vi "Identify Resource Name.vi"() -> ()   [LabVIEW 2010]
doc: "I. Description:\nThis example demonstrates how to acquire a finite amount of data (waveform) using the DAQ device's internal clock.\n\nII. Instructions for Running:\n1. Select the physical channel to correspond to where your signal is input on the DAQ device.\n2. Enter the minimum and maximum voltages.\nNote: For better accuracy try to match the input range to the expected voltage level of the measured signal.\n3. Select the number of samples to acquire.\n4. Set the rate of the acquisition\nNote: The rate should be AT LEAST twice as fast as the maximum frequency component of the signal being acquired.\n\nIII. Block Diagram Steps:\n1. Create an analog input voltage channel.\n2. Set the rate for the sample clock. Additionally, define the sample mode to be finite and set the number of samples to be acquired per channel.\n3. Call the Start VI to start the acquisition.\n4. Use the Read VI to measure multiple samples from N Channels on the device. Set a timeout so an error is returned if the samples are not returned in the specified time limit\n5. Call the Clear Task VI to clear the Task.\n6. Use the popup dialog box to display an error if any.\n \nIV. I/O Connections Overview:\nMake sure your signal input terminal matches the Physical Channel I/O Control. For further connection information, refer to your hardware reference manual."
uses:
  <vilib>/Utility/error.llb/DialogType.ctl
  <vilib>/DAQmx/read.llb/DAQmx Read (Analog 1D Wfm NChan NSamp).vi
  <vilib>/DAQmx/create/channels.llb/DAQmx Create Channel (AI-Voltage-Basic).vi
  <vilib>/DAQmx/configure/timing.llb/DAQmx Timing (Sample Clock).vi
  <vilib>/daqmx/miscellaneous.llb/DAQmx Fill In Error Info.vi
  Program Files/National Instruments/LabVIEW 2010/resource/objmgr/daqmx.rc
panel:
  in  "Desired Channels":string="/ai0:3"
  in  "ProductType you are looking for":string="PXI-4472"
  out "Physical Channels":string
  out "DAQmx Device Name":tag
  out "Array 2":string[](array[string])
  out "DevNames":tag[](array[tag])
  in  "Maximum Value":dbl=10.0 format="%0.2f"
  in  "Minimum Value":dbl=-10.0 format="%0.2f"
  in  "Rate":dbl=10000.0 caption="Sample Rate (Hz)" format="%0.2f"
  in  "Samples per Channel":i32=1000
  out "Measurement":waveform(dbl)[](graph)
  # "For instructions, select Help>>Show Context Help"
  # "e.g. USB-6009"
  # "Device Name of the desired Device\ne.g. Dev1"
  # "These are the channels that you want \nto acquire on. These are concatenated\nwith the device name and must therefore\nstart with a \"/\"\ne.g. /ai0:3"
  # "Channel Parameters"
  # "This is an indicator.\nIt is the result of \nthe name configured\nin the box above"
  # "Timing Parameters"
  # "All device names\npresent in the \nsystem, should\nlook like MAX's\nDAQmx Devices\nlist"
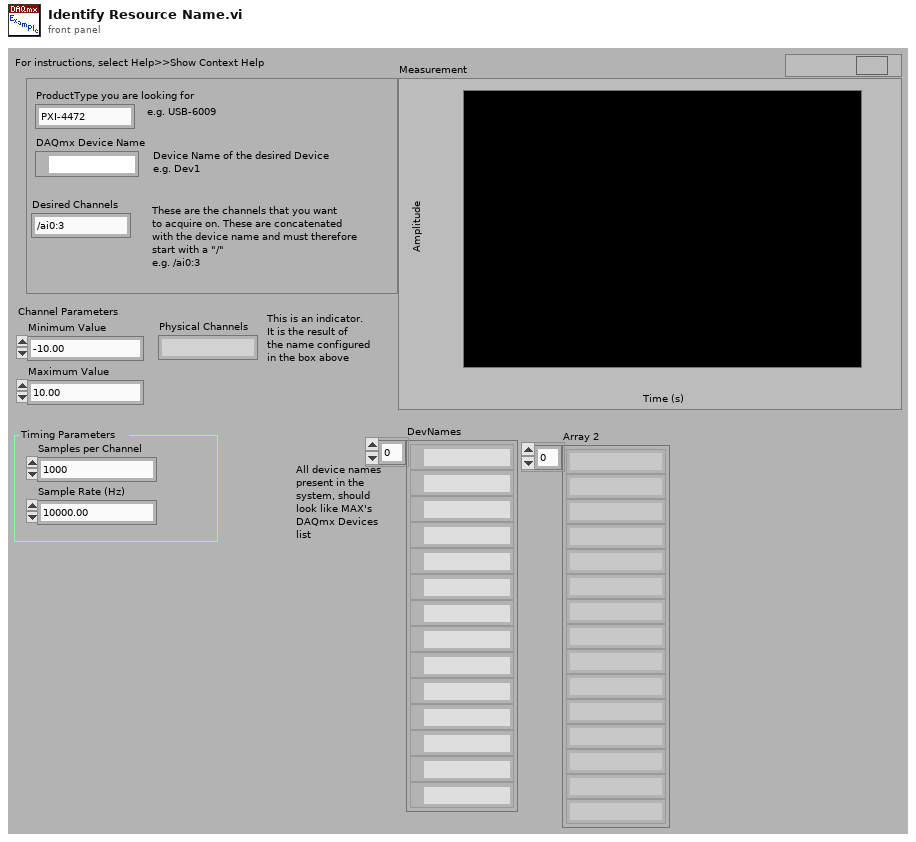
[diagram p1: front panel]
types:
  T1 = typedef "DialogType.ctl" = u16
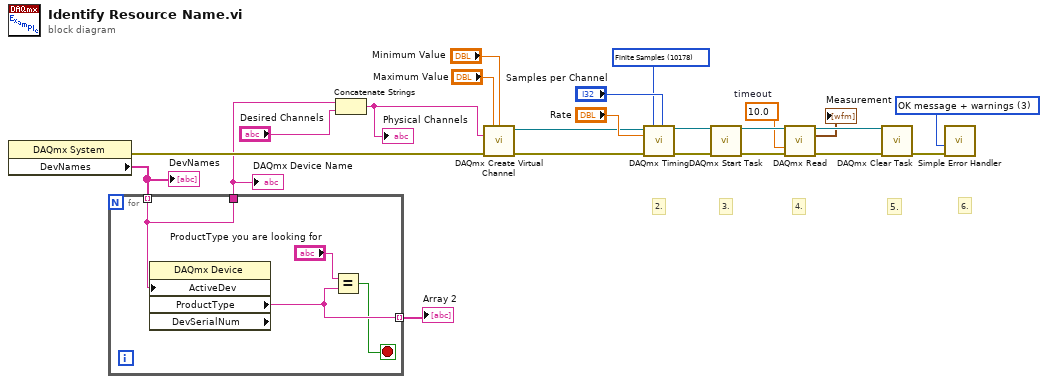
[diagram p0: block diagram]
diagram:
  w8 = T1 3 items=["no dialog", "OK message", "continue or stop message", "OK message + warnings", "continue/stop + warnings"] ("type of dialog (OK msg:1)")
  w9 = 10.0  # timeout
  w14 = 10178 items=["Finite Samples"=10178, "Continuous Samples"=10123] ("sample mode")
  # "6."
  # "5."
  # "3."
  # "4."
  # "2."
  n1 = property class="DAQmx System"() -> (error out=w6:errorcluster, "DevNames"=w5:tag[])  [unwired: 2 in, 1 out]
  "DevNames" <- w5
  n2 = for {
    tunnel: w5 -> [w25] mode=indexing
    tunnel: [w27] -> w4 mode=indexing
    tunnel: [w25] -> w3
    stop <- w26 stop-if-true
    n3 = property class="DAQmx Device" props=["ActiveDev", "ProductType", "DevSerialNum"]("ActiveDev"=w25) -> ("ProductType"=w27:string)  [unwired: 2 in, 3 out]
    n4 = Equal?(x="ProductType you are looking for", y=w27) -> (x = y?=w26:bool)
  }
  "Array 2" <- w4
  "DAQmx Device Name" <- w3
  n5 = Concatenate Strings "Concatenate Strings"(w3, "Desired Channels") -> (w1:string)
  "Physical Channels" <- w1
  n6 = call-poly <vilib>:"DAQmx Create Virtual Channel.vi"("maximum value"="Maximum Value", "minimum value"="Minimum Value", "physical channels"=w1, "error in"=w6) -> ("task out"=w7:refnum<k21>, "error out"=w21:errorcluster)  [unwired: 10 in]
  n7 = call-poly <vilib>:"DAQmx Timing.vi"("task/channels in"=w7, "sample mode"=w14, "samples per channel"="Samples per Channel", "rate"="Rate", "error in"=w21) -> ("task out"=w12:refnum<k21>, "error out"=w11:errorcluster)  [unwired: 9 in]
  n8 = call <vilib>:"DAQmx Start Task.vi"("task/channels in"=w12, "error in"=w11) -> ("task out"=w16:refnum<k21>, "error out"=w20:errorcluster)  [unwired: 12 in]
  n9 = call-poly <vilib>:"DAQmx Read.vi"("task/channels in"=w16, "timeout"=w9, "error in"=w20) -> ("task out"=w15:refnum<k21>, "data"=→"Measurement":waveform(dbl)[], "error out"=w10:errorcluster)  [unwired: 10 in]
  n10 = call <vilib>:"DAQmx Clear Task.vi"("task in"=w15, "error in"=w10) -> ("error out"=w18:errorcluster)  [unwired: 13 in]
  n11 = call <vilib>:"Simple Error Handler.vi"("type of dialog (OK msg:1)"=w8, "error in (no error)"=w18) -> ()  [unwired: 3 in, 5 out]
